vi "Start Tester.vi"(8 "error in":errorcluster, 11 "Tester Settings":T2) -> (0 "error out":errorcluster)   [LabVIEW 2024]
uses:
  Shared Modules/CAN Commands Interpreter/XNET Session Settings.ctl
  Modules/Tester Internal Communication/References - Create.vi
  Modules/Tester Internal Communication/Queues - Create.vi
  Modules/Working Mode/Set Working Mode.vi
  Shared Modules/CAN Commands Interpreter/Target Sessions - Create Database.vi
  Shared Modules/CAN Commands Interpreter/Target Sessions - Initialize Output Session.vi
  Shared Modules/CAN Commands Interpreter/Target Sessions - Initialize Input Session.vi
  Shared Modules/CAN Commands Interpreter/Target Sessions - Start Session.vi
  Modules/UI/User Interface Control.lvlib
  Modules/Tester Internal Communication/Tester InterComm.lvlib
  Shared Modules/CAN Commands Interpreter/CAN Commands.lvlib
  Modules/Working Mode/Tester Working Mode.lvlib
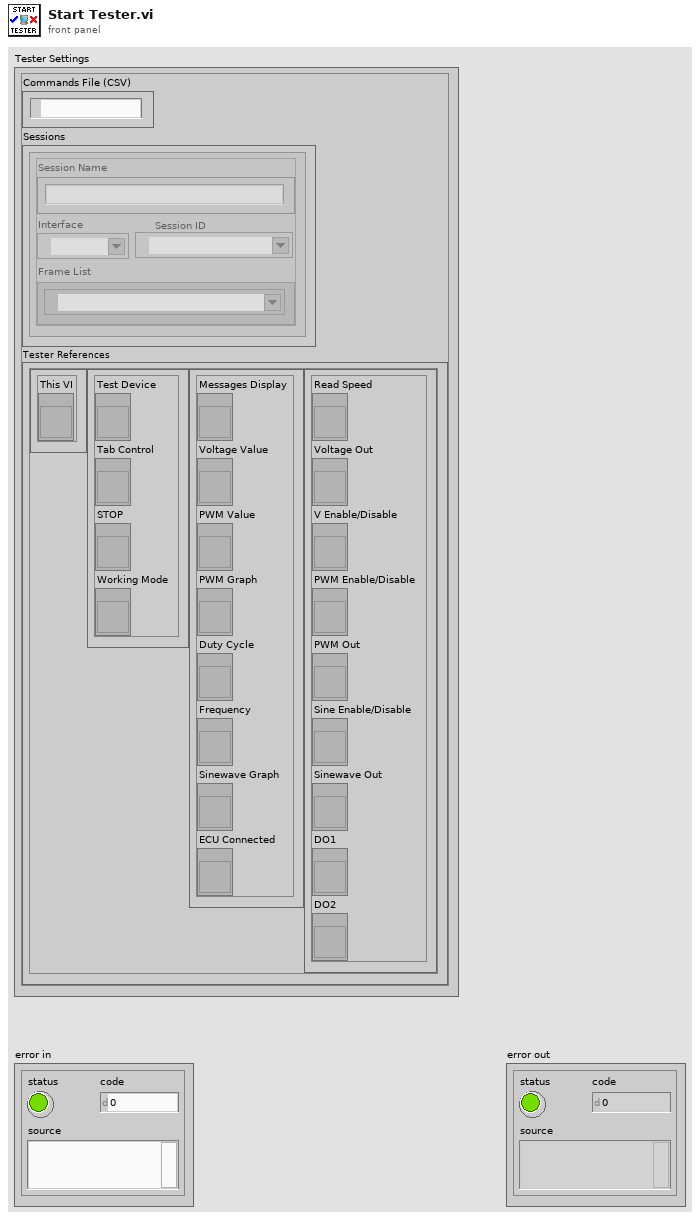
[diagram p1: front panel]
types:
  T1 = typedef "CAN Commands.lvlib/XNET Session Settings.ctl" = cluster{"Interface":refnum<k21>, "Frame List":refnum<k21>[], "Session ID":refnum<k21>, "Session Name":string}
  T2 = cluster{"Commands File (CSV)":path, "Sessions":T1[], "Tester References":cluster{"Cluster":cluster{"This VI":refnum<vi>}, "Cluster":cluster{"Test Device":refnum<vi>, "Tab Control":refnum<vi>, "STOP":refnum<vi>, "Working Mode":refnum<vi>}, "Cluster":cluster{"Messages Display":refnum<vi>, "Voltage Value":refnum<vi>, "PWM Value":refnum<vi>, "PWM Graph":refnum<vi>, "Duty Cycle":refnum<vi>, "Frequency":refnum<vi>, "Sinewave Graph":refnum<vi>, "ECU Connected":refnum<vi>}, "Cluster":cluster{"Read Speed":refnum<vi>, "Voltage Out":refnum<vi>, "V Enable/Disable":refnum<vi>, "PWM Enable/Disable":refnum<vi>, "PWM Out":refnum<vi>, "Sine Enable/Disable":refnum<vi>, "Sinewave Out":refnum<vi>, "DO1":refnum<vi>, "DO2":refnum<vi>}}}
  T3 = cluster{"Cluster":cluster{"This VI":refnum<vi>}, "Cluster":cluster{"Test Device":refnum<vi>, "Tab Control":refnum<vi>, "STOP":refnum<vi>, "Working Mode":refnum<vi>}, "Cluster":cluster{"Messages Display":refnum<vi>, "Voltage Value":refnum<vi>, "PWM Value":refnum<vi>, "PWM Graph":refnum<vi>, "Duty Cycle":refnum<vi>, "Frequency":refnum<vi>, "Sinewave Graph":refnum<vi>, "ECU Connected":refnum<vi>}, "Cluster":cluster{"Read Speed":refnum<vi>, "Voltage Out":refnum<vi>, "V Enable/Disable":refnum<vi>, "PWM Enable/Disable":refnum<vi>, "PWM Out":refnum<vi>, "Sine Enable/Disable":refnum<vi>, "Sinewave Out":refnum<vi>, "DO1":refnum<vi>, "DO2":refnum<vi>}}
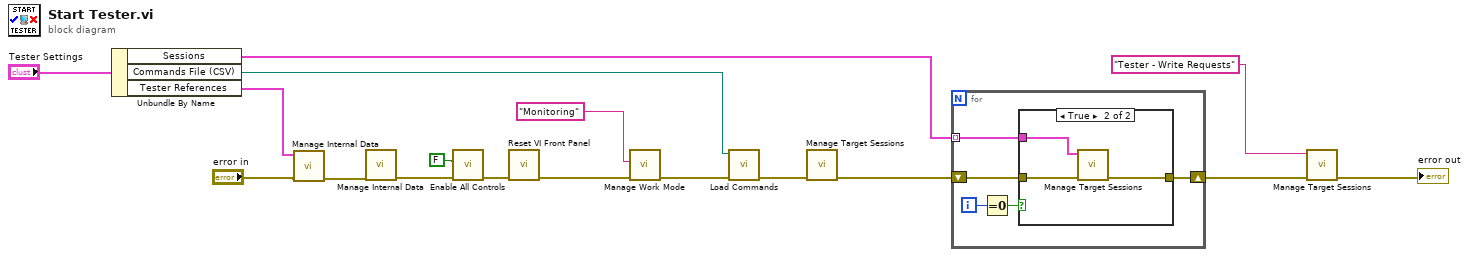
[diagram p0: block diagram]
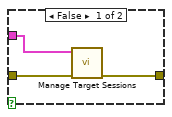
[diagram p2: hidden frame]
diagram:
  n1 = Unbundle By Name("Tester Settings") -> ("Sessions"=w7:T1[], "Commands File (CSV)"=w13:path, "Tester References"=w12:T3)
  n2 = call-poly "Manage Internal Data.vi"("error in"="error in", "References In"=w12) -> ("error out"=w15:errorcluster)  [unwired: 9 in]
  n3 = call-poly "Manage Internal Data.vi"("error in"=w15) -> ("error out"=w4:errorcluster)  [unwired: 10 in]
  n4 = call "Enable All Controls.vi"("error in"=w4, "Enable Controls"=FALSE) -> ("error out"=w16:errorcluster)  [unwired: 9 in]
  n5 = call "Reset VI Front Panel.vi"("error in"=w16) -> ("error out"=w3:errorcluster)  [unwired: 10 in]
  n6 = call-poly "Manage Work Mode.vi"("error in"=w3, "Message"="Monitoring") -> ("error out"=w2:errorcluster)  [unwired: 9 in]
  n7 = call "Load Commands.vi"("error in"=w2, "Commands File (CSV)"=w13) -> ("error out"=w11:errorcluster)  [unwired: 9 in]
  n8 = call-poly "Manage Target Sessions.vi"("error in"=w11) -> ("error out"=w8:errorcluster)  [unwired: 10 in]
  n9 = for {
    shift-right: [w22] -> w9
    shift-left: w8 -> [w21]
    tunnel: w7 -> [w20] mode=indexing
    i -> [w18]
    n10 = Equal To 0?(x=w18) -> (x = 0?=w19:bool)
    n11 = case shown="True" w19 {
      tunnel: [w24 w28] -> w22
      tunnel: w21 -> [w25 w27]
      tunnel: w20 -> [w23 w26]
      frame False {
        n12 = call-poly "Manage Target Sessions.vi"("error in"=w25, "XNET Session Resouces"=w23) -> ("error out"=w24:errorcluster)  [unwired: 9 in]
      }
      frame True {
        n13 = call-poly "Manage Target Sessions.vi"("error in"=w27, "XNET Session Resouces"=w26) -> ("error out"=w28:errorcluster)  [unwired: 9 in]
      }
    }
  }
  n14 = call-poly "Manage Target Sessions.vi"("error in"=w9, "Session Name"="Tester - Write Requests") -> ("error out"=→"error out":errorcluster)  [unwired: 9 in]
